vi "sint32 encode.vi"(11 "sint32":i32) -> (3 "zigzag32":u32)   [LabVIEW 2013, in "protocol buffers encoder.lvlib"]
uses:
  protocol buffers encoder.lvlib
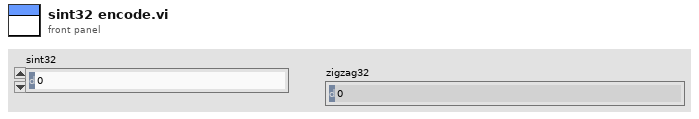
[diagram p1: front panel]
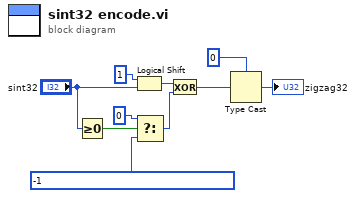
[diagram p0: block diagram]
diagram:
  n1 = Greater Or Equal To 0?(x="sint32") -> (x >= 0?=w10:bool)
  n2 = Logical Shift(y=i16 1, x="sint32") -> (x << y=w7:i32)
  n3 = Select(t=0, s=w10, f=-1 ("y")) -> (s? t:f=w8:i32)
  n4 = Exclusive Or(1:w8, 2:w7) -> (0:w5:i32)
  n5 = Type Cast(type=u32 0 ("y"), x=w5) -> (*(type *) &x=→"zigzag32":u32)
